vi "BH Druck PACE Series In Limits Measurements.vi"() -> ()   [LabVIEW 2022 SP3]
uses:
  <vilib>/Utility/error.llb/DialogType.ctl
  BH Druck PACE Series.lvclass
panel:
  out "Driver Revision":string
  out "Firmware Revision":string
  out "Serial Number":string
  out "Model":string
  out "Manufacturer":string
  in  "Manual Tare Offset":dbl
  in  "Enable Tare (Off)":bool
  in  "Tare Source (0: Auto)":enum16{"Auto", "Manual"}(ring)=enum."Manual"
  in  "In Limits Time (second) (1)":i32=1 min=1 max=60 step=1
  in  "In Limits (%FS) (0.01)":dbl=0.01 min=0.0 max=10.0 step=0.001
  in  "Serial Configuration":T1={"Baud Rate"=9600, "Parity"=0, "Data Bits"=8, "Stop Bits"=10, "Flow Control"=0} {"Flow Control" items=["None", "XON/XOFF", "RTS/CTS", "XON/XOFF & RTS/CTS", "DTR/DSR", "XON/XOFF & DTR/DSR"]; "Stop Bits" items=["1.0"=10, "1.5"=15, "2.0"=20]; "Data Bits" items=["7"=7, "8"=8]; "Parity" items=["None", "Odd", "Even", "Mark", "Space"]; "Baud Rate" items=["300"=300, "600"=600, "1200"=1200, "2400"=2400, "4800"=4800, "9600"=9600, "19200"=19200]}
  in  "Channel (0: Channel A)":u16(ring) items=["Channel A", "Channel B"]
  in  "VISA resource name":refnum<visa-resource-name>
  # "(c)2010-2020  BH Druck  Druck Ltd.  ALL RIGHTS RESERVED."
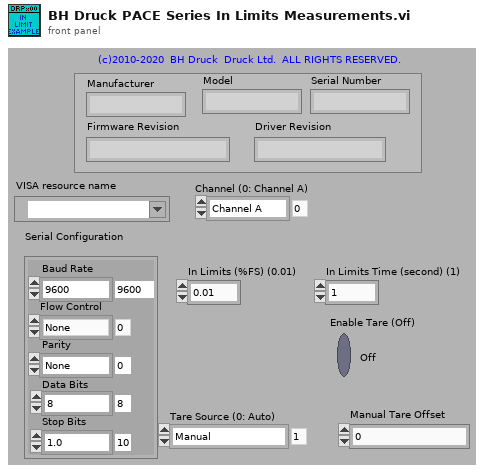
[diagram p1: front panel]
types:
  T1 = cluster{"Baud Rate":u32, "Parity":u16, "Data Bits":u16, "Stop Bits":u16, "Flow Control":u16}
  T2 = typedef "DialogType.ctl" = u16
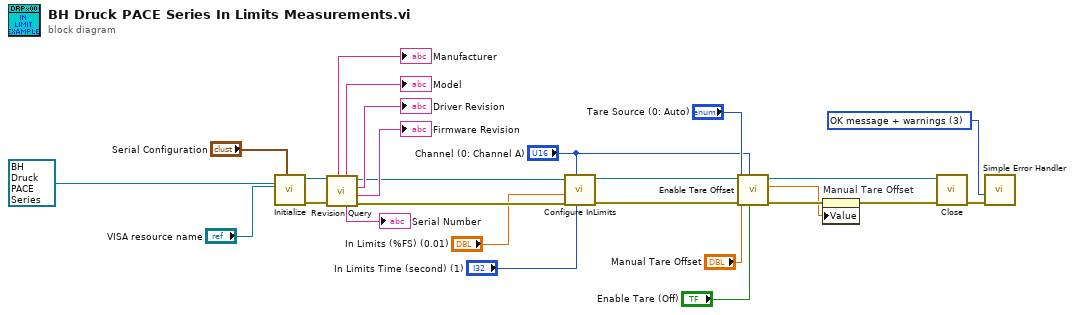
[diagram p0: block diagram]
diagram:
  w15 = T2 3 items=["no dialog", "OK message", "continue or stop message", "OK message + warnings", "continue/stop + warnings"] ("type of dialog (OK msg:1)")
  n1 = call-dynamic "Initialize.vi"("Serial Configuration"="Serial Configuration", "VISA resource name"="VISA resource name", "BH Druck PACE Series in"=refnum<class "BH Druck PACE Series.lvclass"> refnum) -> ("error out"=w24:errorcluster, "BH Druck PACE Series out"=w25:refnum<class "BH Druck PACE Series.lvclass">)  [unwired: 6 in]
  n2 = call-dynamic "Revision Query.vi"("error in (no error)"=w24, "BH Druck PACE Series in"=w25) -> ("error out"=w18:errorcluster, "Firmware Revision"=→"Firmware Revision":string, "Driver Revision"=→"Driver Revision":string, "BH Druck PACE Series out"=w17:refnum<class "BH Druck PACE Series.lvclass">, "Serial Number"=→"Serial Number":string, "Model"=→"Model":string, "Manufacturer"=→"Manufacturer":string)  [unwired: 3 in]
  n3 = call-dynamic "Configure InLimits.vi"("In Limits Time (second) (1)"="In Limits Time (second) (1)", "Channel (0: Channel A)"="Channel (0: Channel A)", "error in (no error)"=w18, "In Limits (%FS) (0.01)"="In Limits (%FS) (0.01)", "BH Druck PACE Series in"=w17) -> ("error out"=w2:errorcluster, "BH Druck PACE Series out"=w3:refnum<class "BH Druck PACE Series.lvclass">)  [unwired: 5 in]
  n4 = call-dynamic "Enable Tare Offset.vi"("Enable Tare (Off)"="Enable Tare (Off)", "Channel (0: Channel A)"="Channel (0: Channel A)", "error in (no error)"=w2, "Manual Tare Offset"="Manual Tare Offset", "Tare Source (0: Auto)"="Tare Source (0: Auto)", "BH Druck PACE Series in"=w3) -> ("error out"=w7:errorcluster, "Tare Offset"=w6:dbl, "BH Druck PACE Series out"=w11:refnum<class "BH Druck PACE Series.lvclass">)  [unwired: 3 in]
  n5 = property on="Manual Tare Offset" class="DigNum (strict)"(error in=w7, "Value"=w6) -> (error out=w5:errorcluster)  [unwired: 1 in, 1 out]
  n6 = call "Close.vi"("error in (no error)"=w5, "BH Druck PACE Series in"=w11) -> ("error out"=w16:errorcluster)  [unwired: 8 in, 1 out]
  n7 = call <vilib>:"Simple Error Handler.vi"("type of dialog (OK msg:1)"=w15, "error in (no error)"=w16) -> ()  [unwired: 3 in, 5 out]
